vi "_hmp4000 Default Instrument Setup.vi"(0 "VISA resource name":refnum<visa-resource-name>, 11 "error in (no error)":errorcluster) -> (4 "VISA resource name out":refnum<visa-resource-name>, 15 "error out":errorcluster)   [LabVIEW 2022 SP3]
doc: "This Utility VI sends a default command string to the instrument whenever a new VISA session is opened, or the instrument is reset.\nThis VI is intended to be used as a subVI for the Initialize.vi and Reset VI. Altering this VI could cause these two VI's to operate incorrectly."
uses:
  hmp4000_rsidr_core.lvlib
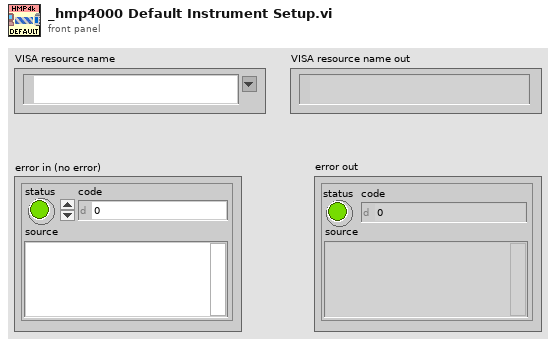
[diagram p1: front panel]
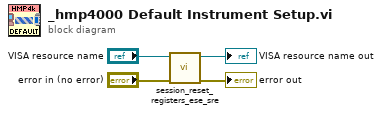
[diagram p0: block diagram]
diagram:
  n1 = call "session_reset_registers_ese_sre.vi"("error in"="error in (no error)", "VISA resource name"="VISA resource name") -> ("error out"=→"error out":errorcluster, "VISA resource name out"=→"VISA resource name out":refnum<visa-resource-name>)  [unwired: 8 in]
